vi "rpm to mm_sec conversion.vi"(8 "error in (no error)":errorcluster, 9 "Final Speed (RPM)":dbl=1.0 min=0.1 max=3000.0 step=0.1 format="%.1f", 10 "Wear Track Diameter":dbl=1.0 min=0.001 max=4.0 step=0.001 format="%.3f", 11 "Initial Speed (RPM)":dbl=100.0 min=0.1 max=3000.0 step=0.1 format="%.1f") -> (0 "error out":errorcluster, 2 "Enter the Final Velocity (m/s) 4":dbl=1.0 min=0.001 max=2.0 step=0.001 format="%.3f", 3 "Enter initial Velocity (m/s)  4":dbl=2.0 min=0.001 max=2.0 step=0.001 format="%.3f")   [LabVIEW 2025]
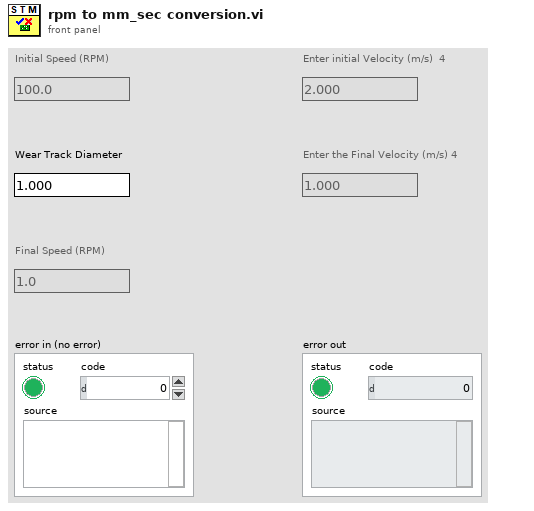
[diagram p1: front panel]
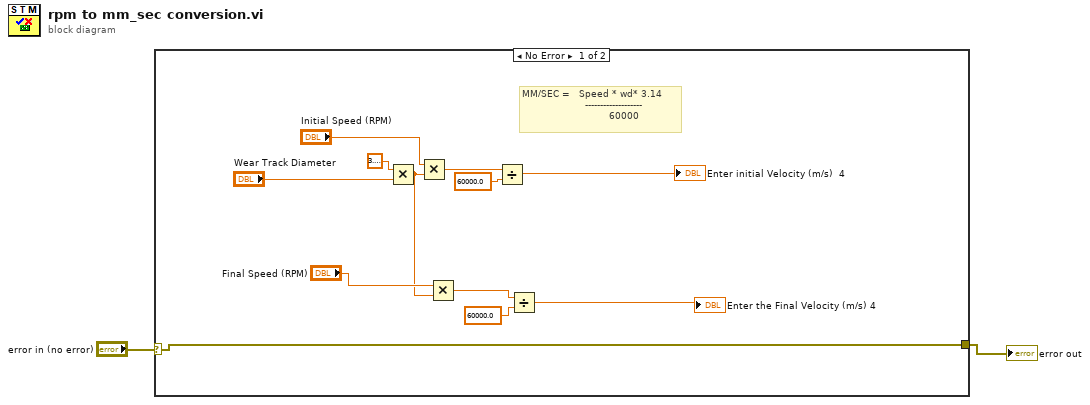
[diagram p0: block diagram]
diagram:
  n1 = case shown="No Error" "error in (no error)" {
    selector: "error in (no error)" -> [w3 _]
    tunnel: [w3 _] -> w2
    frame No Error {
      # "MM/SEC =   Speed * wd* 3.14\n                     -------------------\n                             60000"
      n2 = Multiply(x=3.141592653589793, y="Wear Track Diameter") -> (x*y=w7:dbl)
      n3 = Multiply(x="Initial Speed (RPM)", y=w7) -> (x*y=w11:dbl)
      n4 = Multiply(x="Final Speed (RPM)", y=w7) -> (x*y=w5:dbl)
      n5 = Divide(x=w11, y=60000.0 ("x")) -> (x/y=→"Enter initial Velocity (m/s)  4":dbl)
      n6 = Divide(x=w5, y=60000.0 ("x")) -> (x/y=→"Enter the Final Velocity (m/s) 4":dbl)
    }
    frame Error {
    }
  }
  "error out" <- w2
